vi "Ramsete.vi"() -> ()   [LabVIEW 2023]
uses:
  <vilib>/Analysis/baseanly.llb/Real A x B.vi
  <vilib>/Analysis/_algsub.llb/Vector Norm.vi
  <vilib>/Analysis/_algsub.llb/Real Vector Norm.vi
  <vilib>/Analysis/baseanly.llb/Outer Product.vi
  <vilib>/Analysis/baseanly.llb/Real Outer Product.vi
  <vilib>/robotics/Kinematics/Create Lie Group Matrix.vi
  <vilib>/Analysis/Matrix/Numeric/Conversions/Array To Matrix - RA.vi
  <vilib>/Analysis/7linalg.llb/Create Special Matrix.vi
  <vilib>/Analysis/7linalg.llb/Create Special Real Matrix.vi
  <vilib>/Analysis/Matrix/Numeric/Multiply/Multiply.vi
  <vilib>/Analysis/Matrix/Numeric/Multiply/Multiply - RM,R.vi
  <vilib>/Analysis/Matrix/Numeric/Multiply/Multiply - R,RM.vi
  <vilib>/Analysis/Matrix/Numeric/Add/Add.vi
  <vilib>/Analysis/Matrix/Numeric/Add/Add - RM,RM.vi
  <vilib>/Analysis/Matrix/Numeric/Conversions/Matrix To Array - RM.vi
  <vilib>/Analysis/NI_AALBase.lvlib
  <vilib>/robotics/Kinematics/NI_Kinematics.lvlib
  <vilib>/Analysis/Matrix/NI_Matrix.lvlib
panel:
  in  "omega_d":dbl
  in  "v_d":dbl
  in  "output cluster 2":cluster{dbl, dbl, dbl}
  in  "output cluster":cluster{dbl, dbl, dbl}
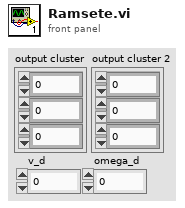
[diagram p1: front panel]
types:
  T1 = typedef "NI_Matrix.lvlib/RealMatrix.ctl" = dbl[][]
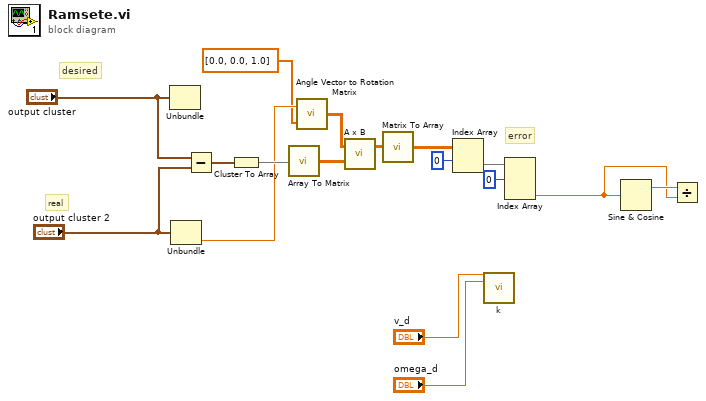
[diagram p0: block diagram]
diagram:
  # "error"
  # "desired"
  # "real"
  n1 = Unbundle("output cluster") -> ()  [unwired: 3 out]
  n2 = Unbundle("output cluster 2") -> (w11:dbl)  [unwired: 2 out]
  n3 = Subtract(x="output cluster", y="output cluster 2") -> (x-y=w15:cluster{dbl, dbl, dbl})
  n4 = Cluster To Array(cluster=w15) -> (array=w14:dbl[])
  n5 = call-poly <vilib>:"Array To Matrix.vi"("Real 1D Array"=w14) -> ("Real Matrix (Column Vector)"=w13:T1)
  n6 = call <vilib>:"Angle Vector to Rotation Matrix.vi"("vector"=dbl[] [0.0, 0.0, 1.0], "angle"=w11) -> ("rotation matrix"=w12:T1)
  n7 = call-poly <vilib>:"A x B.vi"("B"=w13, "A"=w12) -> ("A x B"=w9:T1)  [unwired: 1 out]
  n8 = call-poly <vilib>:"Matrix To Array.vi"("Real Matrix"=w9) -> ("Real 2D Array"=w8:dbl[][])
  n9 = Index Array(array=w8, index (row)=0) -> (element=w6:dbl[])  [unwired: 1 in]
  n10 = call "k.vi"("omega_d"="omega_d", "v_d"="v_d") -> ()  [unwired: 9 in, 1 out]
  n11 = Index Array(array=w6, index #1=0 ("index")) -> (element #3=w3:dbl)  [unwired: 2 in, 2 out]
  n12 = Sine & Cosine(0:w3) -> (1:w4:dbl)  [unwired: 1 out]
  n13 = Divide(x=w4, y=w3) -> ()  [unwired: 1 out]
